vi "GL_SetVandA.vi"(8 "error in":errorcluster, 9 "ByPass Pop up?":bool, 10 "Motion Settings":T1 {"3rd Axis" items=["x", "y", "z", "w"]; "Xtra planes" min=1; "Xtra plane\ndistance  (um)" min=0; "Distance between\nscan planes (um)" format="%.2f"; "Distance between\nscan lines (um)" format="%.2f"; "SMAC Axis" items=["None"=0, "Axis 1"=1, "Axis 2"=2, "Axis 3"=3, "Axis 4"=4, "Axis 5"=5, "Axis 6"=6, "Axis 7"=7, "Axis 8"=8, "Vector Space 1"=17, "Vector Space 2"=18, "Vector Space 3"=19, "Vector Space 4"=20]; "Motion Bd ID" min=1 max=32 step=1}, 11 "Refnum in":refnum<k7>) -> (0 "error out":errorcluster, 2 "Motion Settings Out":T1 {"3rd Axis" items=["x", "y", "z", "w"]; "Xtra planes" min=1; "Xtra plane\ndistance  (um)" min=0; "Distance between\nscan planes (um)" format="%.2f"; "Distance between\nscan lines (um)" format="%.2f"; "SMAC Axis" items=["None"=0, "Axis 1"=1, "Axis 2"=2, "Axis 3"=3, "Axis 4"=4, "Axis 5"=5, "Axis 6"=6, "Axis 7"=7, "Axis 8"=8, "Vector Space 1"=17, "Vector Space 2"=18, "Vector Space 3"=19, "Vector Space 4"=20]; "Motion Bd ID" min=1 max=32 step=1}, 3 "ref out":refnum<k7>)   [LabVIEW 2022 SP3]
uses:
  NI_controller/-NI_MotionRoutines/MotionParameters.ctl
  NI_controller/-NI_MotionRoutines/MotionSys.ctl
  -MotionRoutines/ScanAxis.ctl
  -MotionRoutines/3rdAxis.ctl
  Command Menu.ctl
panel:
  # "1-D and 2-D B scan settings"
  # "1-D and 2-D B scan settings"
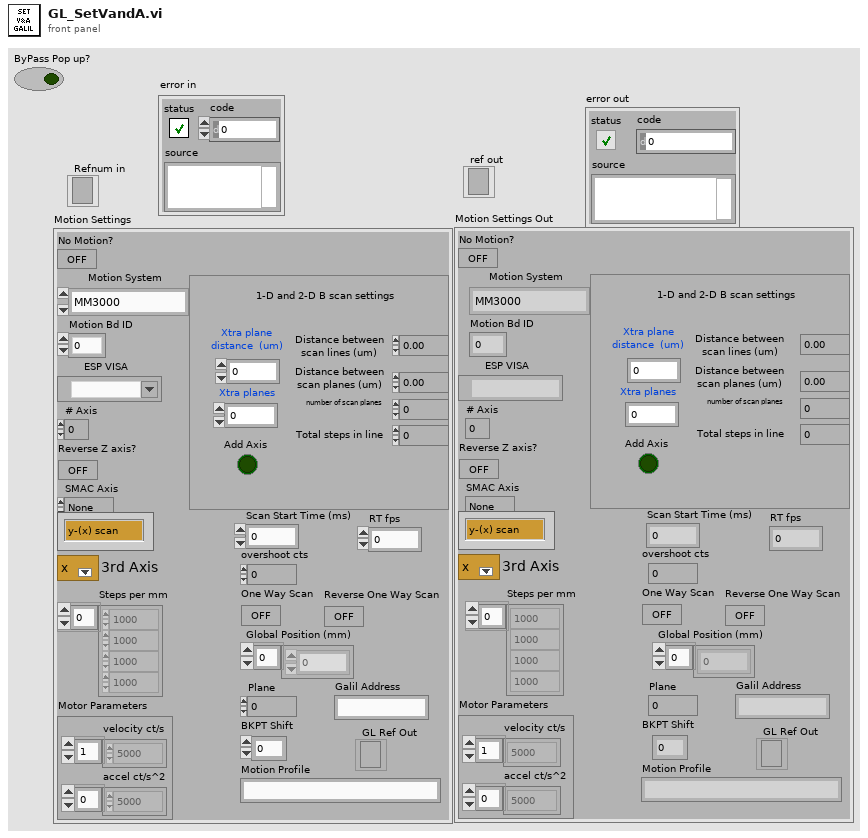
[diagram p1: front panel]
types:
  T1 = typedef "MotionParameters.ctl" = cluster{"No Motion?":bool, "Motion System":T2, "Motion Bd ID":u8, "Motion Profile":string, "# Axis":i8, "Reverse Z axis?":bool, "SMAC Axis":u16, "scan pair":T3, "RT fps":sgl, "Steps per mm":i32[], "Motor Parameters":cluster{"velocity ct/s":dbl[], "accel ct/s^2":dbl[]}, "One Way Scan":bool, "Reverse One Way Scan":bool, "Global Position (mm)":dbl[], "Plane":i32, "Distance between\nscan lines (um)":sgl, "Distance between\nscan planes (um)":sgl, "number of scan planes":i32, "Total steps in line":i32, "Xtra plane\ndistance  (um)":i32, "Xtra planes ":i32, "Add Axis":bool, "overshoot cts":i32, "BKPT Shift":i32, "Scan Start Time (ms)":u32, "ESP VISA":refnum<visa-resource-name>, "3rd Axis":T4, "GL Ref Out":refnum<k7>, "Galil Address":string}
  T2 = typedef "MotionSys.ctl" = enum16{"MM3000", "NI 735x", "Newport ESP", "No Motion Card", "Galil"}
  T3 = typedef "ScanAxis.ctl" = enum16{"y-(x) scan", "x-(y) scan", "z-(x) scan", "z-(y) scan", "y-(z) scan", "x-(z) scan", "w-(x) scan", "w-(y) scan", "w-(z) scan", "x-(w) scan", "y-(w) scan", "z-(w) scan"}
  T4 = typedef "3rdAxis.ctl" = u16
  T5 = typedef "Command Menu.ctl" = enum16{"CommandPassThrough", "Abort Motion", "Define Pos", "Velocity", "Acceleration", "Deceleration", "Position Rel", "Postion Abs", "Begin Move", "After Move", "Home", "KI", "KD", "KP", "IL", "Config I/O", "Set Bit", "Clear Bit", "Motor Off", "Moto On", "Status", "Execute", "Halt Execute", "HX Status", "Tell Velocity", "Check Motion", "BreakPoint", "Tell Position", "Current Code Line", "Tell Switches", "OC Force On", "OC Off", "Pos Soft Limit", "Rev Soft Limit"}
  T6 = typedef "GL Axis Control.ctl" = u16
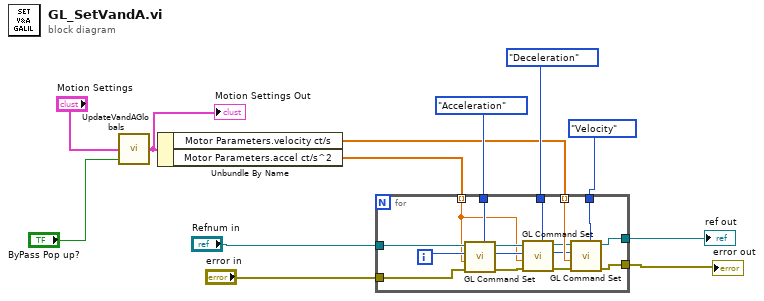
[diagram p0: block diagram]
diagram:
  n1 = call "UpdateVandAGlobals.vi"("ByPass Pop up?"="ByPass Pop up?", "Motion Settings"="Motion Settings") -> ("Motion Settings Out"=w8:T1)  [unwired: 2 in, 1 out]
  "Motion Settings Out" <- w8
  n2 = Unbundle By Name(w8) -> ("Motor Parameters.velocity ct/s"=w6:dbl[], "Motor Parameters.accel ct/s^2"=w4:dbl[])
  n3 = for {
    tunnel: [w27] -> w5
    tunnel: w4 -> [w15] mode=indexing
    tunnel: w6 -> [w26] mode=indexing
    tunnel: "Refnum in" -> [w25]
    tunnel: Command_Menu."Acceleration" ("Command") -> [w24]
    tunnel: Command_Menu."Velocity" ("Command") -> [w23]
    tunnel: Command_Menu."Deceleration" ("Command") -> [w16]
    tunnel: [w14] -> w3
    tunnel: "error in" -> [w13]
    i -> [w28]
    n4 = call "GL Command Set.vi"("Command"=w24, "error in (no error)"=w13, "Value"=w15, "Axis"=w28, "Galil.IGalil"=w25) -> ("error out"=w22:errorcluster, "Axis Out"=w20:T6, "ref out"=w18:refnum<k7>)  [unwired: 2 in, 2 out]
    n5 = call "GL Command Set.vi"("Command"=w16, "error in (no error)"=w22, "Value"=w15, "Axis"=w20, "Galil.IGalil"=w18) -> ("error out"=w21:errorcluster, "Axis Out"=w19:T6, "ref out"=w17:refnum<k7>)  [unwired: 2 in, 2 out]
    n6 = call "GL Command Set.vi"("Command"=w23, "error in (no error)"=w21, "Value"=w26, "Axis"=w19, "Galil.IGalil"=w17) -> ("error out"=w27:errorcluster, "ref out"=w14:refnum<k7>)  [unwired: 2 in, 3 out]
  }
  "error out" <- w5
  "ref out" <- w3
